vi "Insert.vi"(8 "error in (no error)":errorcluster caption="entrée d'erreur (pas d'erreur)", 11 "Database Drivers en entrée":refnum<class "Database Drivers.lvclass">) -> (0 "error out":errorcluster caption="sortie d'erreur", 3 "Database Drivers en sortie":refnum<class "Database Drivers.lvclass">)   [LabVIEW 2020, in "Library Instrument & Equipement.lvlib" / "Library Database.lvlib" / "Database Drivers.lvclass"]
uses:
  Database Drivers.lvclass
  Database Drivers.lvclass/Database Drivers.ctl
  <vilib>/addons/database/NI_Database_API.lvlib
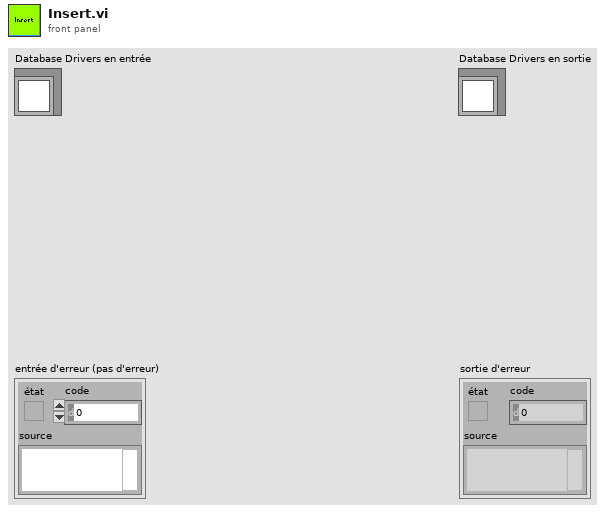
[diagram p1: front panel]
types:
  T1 = typedef "NI_Database_API.lvlib/Conn ObjectReference.ctl" = refnum<k1>
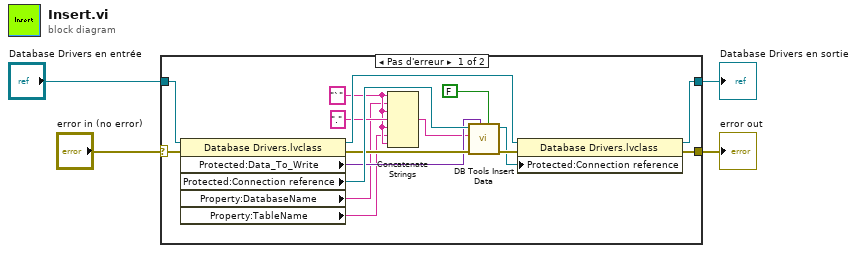
[diagram p0: block diagram]
diagram:
  n1 = case shown="Pas d'erreur" "error in (no error)" {
    selector: "error in (no error)" -> [w16 w22]
    tunnel: [w12 w22] -> w3
    tunnel: [w13 w21] -> w1
    tunnel: "Database Drivers en entrée" -> [w15 w21]
    frame No Error {
      w8 = "`" ("chaîne")
      n2 = property class="Database Drivers.lvclass"(reference=w15, error in=w16) -> (reference out=w10:refnum<class "Database Drivers.lvclass">, error out=w19:errorcluster, "Protected:Data_To_Write"=w17:variant, "Protected:Connection reference"=w20:T1, "Property:DatabaseName"=w7:string, "Property:TableName"=w6:string)
      n3 = Concatenate Strings(w8, w7, w8, "." ("chaîne"), w8, w6, w8) -> (w5:string)
      n4 = call <vilib>:"DB Tools Insert Data.vi"("create table? (F)"=FALSE, "data"=w17, "error in (no error)"=w19, "table"=w5, "connection reference"=w20) -> ("error out"=w14:errorcluster, "connection reference out"=w11:T1)  [unwired: 5 in]
      n5 = property class="Database Drivers.lvclass"(reference=w10, error in=w14, "Protected:Connection reference"=w11) -> (reference out=w13:refnum<class "Database Drivers.lvclass">, error out=w12:errorcluster)
    }
    frame Error {
    }
  }
  "error out" <- w3
  "Database Drivers en sortie" <- w1
